vi "get_settings_cluster.vi"(8 "error in (no error)":errorcluster, 11 "GenericPlugin in":refnum<class "StringGeneratorAK110125StimServerCmd.lvclass">) -> (0 "error out":errorcluster, 2 "settings cluster":variant, 3 "GenericPlugin out":refnum<class "StringGeneratorAK110125StimServerCmd.lvclass">)   [LabVIEW 2010, in "StringGeneratorAK110125StimServerCmd.lvclass"]
uses:
  StringGeneratorAK110125StimServerCmd.lvclass
  GenericStringGenerator/GenericStringGenerator/GenericStringGenerator.lvclass
  StringGeneratorAK110125StimServerCmd.lvclass/StringGeneratorAK110125StimServerCmd.ctl
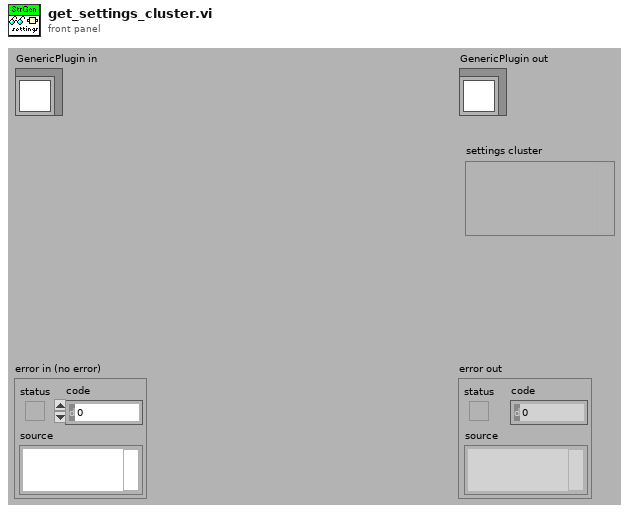
[diagram p1: front panel]
types:
  T1 = cluster{"stimulus IDs with spaces":string, "stimulus":string, "blank time (s)":string, "randomize":bool, "user sequence":bool}
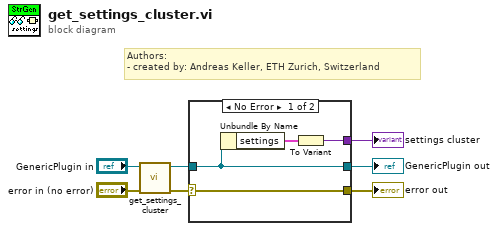
[diagram p0: block diagram]
diagram:
  # "Authors: \n- created by: Andreas Keller, ETH Zurich, Switzerland"
  n1 = call-parent "get_settings_cluster.vi"("error in (no error)"="error in (no error)", "GenericPlugin in"="GenericPlugin in") -> ("error out"=w5:errorcluster, "GenericPlugin out"=w3:refnum<class "StringGeneratorAK110125StimServerCmd.lvclass">)  [unwired: 7 in, 1 out]
  n2 = case shown="No Error" w5 {
    selector: w5 -> [w11 w13]
    tunnel: [w11 w13] -> w4
    tunnel: [w10 w12] -> w2
    tunnel: w3 -> [w10 w12]
    tunnel: [w8 _] -> w1
    frame No Error {
      n3 = Unbundle By Name(w10) -> ("settings"=w9:T1)
      n4 = To Variant(anything=w9) -> (Variant=w8:variant)
    }
    frame Error {
    }
  }
  "error out" <- w4
  "GenericPlugin out" <- w2
  "settings cluster" <- w1
